vi "dfd_DA SRate Handshaking Dummy.vi"(11 "input valid":bool=TRUE) -> (0 "last bit":bool=TRUE, 1 "shift enable":bool=TRUE, 2 "load":bool=TRUE, 3 "ready for input":bool=TRUE)   [LabVIEW 2017]
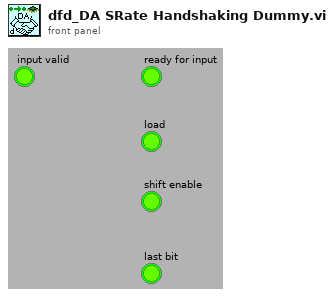
[diagram p1: front panel]
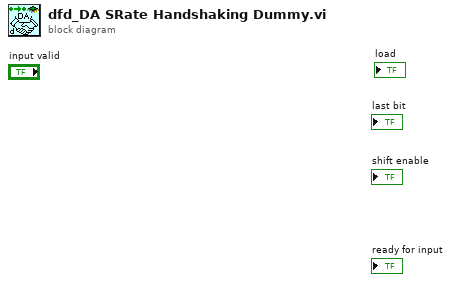
[diagram p0: block diagram]
diagram:
